vi "SentinelController v33.vi"() -> ()   [LabVIEW 2011] (continued)
                                n1247 = local write "SC handler states hid"(SC_handler_states."responding to serial poll" ("SC Test Interface States")) -> ()
                                }
                                }
                                }
                                }
                              }
                              frame "reading" {
                                n1248 = flat-sequence {
                                tunnel: [w1473] -> w1470
                                tunnel: w1470 -> [w1486]
                                tunnel: [w1486] -> w1469
                                tunnel: w1469 -> [w1489]
                                tunnel: [w1488] -> w1468
                                tunnel: w1468 -> [w1490]
                                frame #0 {
                                n1249 = local read "VISA bus 0 resource name out hid"() -> (w1479:refnum<visa-resource-name>)
                                n1250 = local read "VISA bus 0 error out hid"() -> (w1480:errorcluster)
                                n1251 = local read "GPIB Bus 0 traffic"() -> (w1477:string)
                                n1252 = VISA Read(VISA resource name=w1479, byte count=256, error in (no error)=w1480) -> (VISA resource name out=w1478:refnum<visa-resource-name>, read buffer=w1473:string, error out=w1481:errorcluster)  [unwired: 1 out]
                                n1253 = String Subset(string=w1473, length (rest)=1 ("length (rest)")) -> ()  [unwired: 1 in, 1 out]
                                n1254 = local write "VISA bus 0 resource name out hid"(w1478) -> ()
                                n1255 = local write "Message from tester hid"(w1473) -> ()
                                n1256 = Unbundle By Name(w1481) -> ("status"=w1484:bool)
                                n1257 = Concatenate Strings(w1477, "\r\n", "Bus 0 read: " ("string"), w1473) -> (w1475:string)
                                n1258 = local write "GPIB Bus 0 traffic"(w1475) -> ()
                                n1259 = local write "GPIB bus 0 read error"(w1484) -> ()
                                }
                                frame #1 {
                                n1260 = local read "Slow for  Diagnostics"() -> (w1485:bool)
                                n1261 = case shown="True" w1485 {
                                frame False {
                                }
                                frame True {
                                n1262 = local read "GPIB wait time (ms)"() -> (w1487:u32)
                                n1263 = Wait (ms)(milliseconds to wait=w1487) -> ()  [unwired: 1 out]
                                }
                                }
                                }
                                frame #2 {
                                n1264 = call <vilib>:"Trim Whitespace.vi"("string"=w1489) -> ("trimmed string"=w1488:string)  [unwired: 1 in]
                                }
                                frame #3 {
                                n1265 = Match Pattern(string=w1490, regular expression="?") -> (offset past match=w1493:i32)  [unwired: 1 in, 3 out]
                                n1266 = Greater Or Equal To 0?(x=w1493) -> (x >= 0?=w1491:bool)
                                n1267 = case shown="False" w1491 {
                                tunnel: w1490 -> [w1497 w1512]
                                frame False {
                                n1268 = Match Pattern(string=w1497, regular expression=":" ("true string")) -> (offset past match=w1494:i32)  [unwired: 1 in, 3 out]
                                n1269 = Greater Or Equal To 0?(x=w1494) -> (x >= 0?=w1495:bool)
                                n1270 = case shown="False" w1495 {
                                tunnel: w1497 -> [w1500 w1507]
                                frame False {
                                n1271 = call <vilib>:"Space Constant.vi"() -> ("String"=w1501:string)
                                n1272 = Match Pattern(string=w1500, regular expression=w1501) -> (offset past match=w1499:i32)  [unwired: 1 in, 3 out]
                                n1273 = Greater Or Equal To 0?(x=w1499) -> (x >= 0?=w1498:bool)
                                n1274 = case shown="False" w1498 {
                                tunnel: w1500 -> [w1502 w1504]
                                frame False {
                                n1275 = local write "GPIB parsed msg from tester hid"(w1502) -> ()
                                }
                                frame True {
                                n1276 = call <vilib>:"Space Constant.vi"() -> ("String"=w1505:string)
                                n1277 = Match Pattern(string=w1504, regular expression=w1505) -> (before substring=w1503:string)  [unwired: 1 in, 3 out]
                                n1278 = local write "GPIB parsed msg from tester hid"(w1503) -> ()
                                }
                                }
                                }
                                frame True {
                                n1279 = Match Pattern(string=w1507, regular expression=":") -> (before substring=w1506:string)  [unwired: 1 in, 3 out]
                                n1280 = local write "GPIB parsed msg from tester hid"(w1506) -> ()
                                }
                                }
                                }
                                frame True {
                                w1510 = "?" ("regular expression")
                                n1281 = Match Pattern(string=w1512, regular expression=w1510) -> (before substring=w1511:string)  [unwired: 1 in, 3 out]
                                n1282 = Concatenate Strings(w1511, w1510) -> (w1509:string)
                                n1283 = local write "GPIB parsed msg from tester hid"(w1509) -> ()
                                }
                                }
                                }
                                frame #4 {
                                n1284 = local read "GPIB parsed msg from tester hid"() -> (w1513:string)
                                n1285 = case shown="\"Fullsites?\"" w1513 {
                                frame "SQR" {
                                n1286 = local write "SC handler states hid"(SC_handler_states."responding to SRQ" ("SC Test Interface States")) -> ()
                                }
                                frame "*IDN?" {
                                n1287 = local write "SC handler states hid"(SC_handler_states."responding to *IDN?" ("SC Test Interface States")) -> ()
                                }
                                frame "FR?" {
                                n1288 = local write "SC handler states hid"(SC_handler_states."responding to FR?" ("SC Test Interface States")) -> ()
                                }
                                frame "*STB?" {
                                n1289 = local write "SC handler states hid"(SC_handler_states."responding to serial poll" ("SC Test Interface States")) -> ()
                                }
                                frame "SITES?" {
                                n1290 = local read "Tester online"() -> (w1520:bool)
                                n1291 = local read "POWER"() -> (w1518:bool)
                                n1292 = Compound Arithmetic op=AND(w1520, w1518) -> (w1519:bool)
                                n1293 = case shown="True" w1519 {
                                frame False {
                                n1294 = local write "SC handler states hid"(SC_handler_states."closing bus" ("SC virtual handler states")) -> ()
                                }
                                frame True {
                                n1295 = flat-sequence {
                                frame #0 {
                                n1296 = while {
                                stop <- w1523 stop-if-true
                                n1297 = local read "H1 Ready with sites"() -> (w1525:bool)
                                n1298 = local read "H2 Ready with sites"() -> (w1524:bool)
                                n1299 = Or(x=w1525, y=w1524) -> (x .or. y?=w1523:bool)
                                n1300 = Wait (ms)(milliseconds to wait=u32 5) -> ()  [unwired: 1 out]
                                }
                                }
                                frame #1 {
                                n1301 = local write "SC handler states hid"(SC_handler_states."responding to serial poll" ("SC Test Interface States")) -> ()
                                }
                                }
                                }
                                }
                                }
                                frame "Fullsites?" {
                                n1302 = local read "Tester online"() -> (w1529:bool)
                                n1303 = local read "POWER"() -> (w1527:bool)
                                n1304 = Compound Arithmetic op=AND(w1529, w1527) -> (w1528:bool)
                                n1305 = case shown="True" w1528 {
                                frame False {
                                n1306 = local write "SC handler states hid"(SC_handler_states."closing bus" ("SC virtual handler states")) -> ()
                                }
                                frame True {
                                n1307 = flat-sequence {
                                frame #0 {
                                n1308 = while {
                                stop <- w1532 stop-if-true
                                n1309 = local read "H1 Lock"() -> (w1534:bool)
                                n1310 = local read "H2 Lock"() -> (w1533:bool)
                                n1311 = Or(x=w1534, y=w1533) -> (x .or. y?=w1532:bool)
                                n1312 = Wait (ms)(milliseconds to wait=u32 5) -> ()  [unwired: 1 out]
                                }
                                }
                                frame #1 {
                                n1313 = local write "SC handler states hid"(SC_handler_states."responding to Fullsites?" ("SC Test Interface States")) -> ()
                                }
                                }
                                }
                                }
                                }
                                frame "HIDN?" {
                                n1314 = local write "SC handler states hid"(SC_handler_states."responding to HIDN?" ("SC Test Interface States")) -> ()
                                }
                                frame "HAND?" {
                                n1315 = local write "SC handler states hid"(SC_handler_states."respond to HAND?" ("SC Test Interface States")) -> ()
                                }
                                frame "A BIN" {
                                n1316 = flat-sequence {
                                frame #0 {
                                n1317 = local read "Message from tester hid"() -> (w1538:string)
                                n1318 = local write "Binning string from tester hid"(w1538) -> ()
                                }
                                frame #1 {
                                n1319 = local write "SC handler states hid"(SC_handler_states."responding to HIDN?" ("SC Test Interface States")) -> ()
                                }
                                }
                                }
                                frame "BINON" {
                                # "THis may need to be handler specific (lock dependent)"
                                n1320 = flat-sequence {
                                frame #0 {
                                n1321 = local read "Message from tester hid"() -> (w1540:string)
                                n1322 = local write "Binning string from tester hid"(w1540) -> ()
                                }
                                frame #1 {
                                n1323 = local write "SC handler states hid"(SC_handler_states."responding to BINON" ("SC Test Interface States")) -> ()
                                }
                                }
                                }
                                frame "ECHOOK" {
                                n1324 = local write "SC handler states hid"(SC_handler_states."responding to ECHOOK" ("SC Test Interface States")) -> ()
                                }
                                frame "ECHONG" {
                                n1325 = local write "SC handler states hid"(SC_handler_states."responding to ECHONG" ("SC Test Interface States")) -> ()
                                }
                                frame Default {
                                n1326 = local write "SC handler states hid"(SC_handler_states."waiting on event" ("SC Test Interface States")) -> ()
                                }
                                }
                                }
                                }
                              }
                              frame "responding to *IDN?" {
                                n1327 = flat-sequence {
                                frame #0 {
                                n1328 = while {
                                stop <- w1548 stop-if-true
                                w1550 = "Sentinel Controller Handler Interface"
                                n1329 = local read "VISA bus 0 resource name out hid"() -> (w1558:refnum<visa-resource-name>)
                                n1330 = local read "VISA bus 0 error out hid"() -> (w1557:errorcluster)
                                n1331 = local read "GPIB Bus 0 traffic"() -> (w1554:string)
                                n1332 = VISA Write(VISA resource name=w1558, write buffer=w1550, error in (no error)=w1557) -> (VISA resource name out=w1556:refnum<visa-resource-name>, return count=w1549:u32, error out=w1555:errorcluster)
                                n1333 = local write "VISA bus 0 resource name out hid"(w1556) -> ()
                                n1334 = local write "VISA bus 0 error out hid"(w1555) -> ()
                                n1335 = Unbundle By Name(w1555) -> ("status"=w1547:bool)
                                n1336 = Concatenate Strings(w1554, "\r\n", "Bus 0 write: " ("string"), w1550) -> (w1552:string)
                                n1337 = Greater Than 0?(x=w1549) -> (x > 0?=w1548:bool)
                                n1338 = local write "GPIB bus 0 write error"(w1547) -> ()
                                n1339 = local write "GPIB Bus 0 traffic"(w1552) -> ()
                                }
                                }
                                frame #1 {
                                n1340 = local write "SC handler states hid"(SC_handler_states."waiting on event" ("SC Test Interface States")) -> ()
                                }
                                }
                              }
                              frame "responding to SRQ" {
                                n1341 = flat-sequence {
                                frame #0 {
                                n1342 = local read "GPIB Bus 0 traffic"() -> (w1566:string)
                                n1343 = Concatenate Strings(w1566, "\r\n", "Bus 0 write: " ("string"), "Responding to \"SRQ MASK 65\" from tester.\nThis message is sent to NS6040 handlers every cycle.\nNo response back to tester.") -> (w1564:string)
                                n1344 = local write "GPIB Bus 0 traffic"(w1564) -> ()
                                }
                                frame #1 {
                                n1345 = local write "SC handler states hid"(SC_handler_states."waiting on event" ("SC Test Interface States")) -> ()
                                }
                                }
                              }
                              frame "respond to HAND?" {
                                n1346 = local read "H1 Lock"() -> (w1570:bool)
                                n1347 = case shown="False" w1570 {
                                frame False {
                                n1348 = local read "H2 Lock"() -> (w1571:bool)
                                n1349 = case shown="True" w1571 {
                                frame False {
                                n1350 = flat-sequence {
                                frame #0 {
                                n1351 = One Button Dialog(message="Fatal error 200:\nThe SC responded to a handler being ready with devices\nto test, but when the SC check for a lock when responding\nto *HAND?, no handler had a lock. \nPlease report this bug to Celerint at www.celerint.com  ") -> ()  [unwired: 1 in, 1 out]
                                }
                                frame #1 {
                                n1352 = local write "SC handler states hid"(SC_handler_states."closing bus" ("SC Test Interface States")) -> ()
                                }
                                }
                                }
                                frame True {
                                n1353 = flat-sequence {
                                frame #0 {
                                n1354 = while {
                                stop <- w1575 stop-if-true
                                w1576 = "H2" ("string")
                                n1355 = local read "VISA bus 0 resource name out hid"() -> (w1582:refnum<visa-resource-name>)
                                n1356 = local read "GPIB Bus 0 traffic"() -> (w1580:string)
                                n1357 = local read "VISA bus 0 error out hid"() -> (w1581:errorcluster)
                                n1358 = Concatenate Strings(w1580, "\r\n", "H2: Bus 0 write: " ("string"), w1576) -> (w1578:string)
                                n1359 = VISA Write(VISA resource name=w1582, write buffer=w1576, error in (no error)=w1581) -> (VISA resource name out=w1583:refnum<visa-resource-name>, return count=w1574:u32, error out=w1584:errorcluster)
                                n1360 = local write "VISA bus 0 error out hid"(w1584) -> ()
                                n1361 = Unbundle By Name(w1584) -> ("status"=w1585:bool)
                                n1362 = local write "GPIB Bus 0 traffic"(w1578) -> ()
                                n1363 = Greater Than 0?(x=w1574) -> (x > 0?=w1575:bool)
                                n1364 = local write "VISA bus 0 resource name out hid"(w1583) -> ()
                                n1365 = local write "GPIB bus 0 write error"(w1585) -> ()
                                }
                                }
                                frame #1 {
                                n1366 = local write "SC handler states hid"(SC_handler_states."waiting on event" ("SC Test Interface States")) -> ()
                                }
                                }
                                }
                                }
                                }
                                frame True {
                                n1367 = flat-sequence {
                                frame #0 {
                                n1368 = while {
                                stop <- w1588 stop-if-true
                                w1589 = "H1" ("string")
                                n1369 = local read "VISA bus 0 resource name out hid"() -> (w1595:refnum<visa-resource-name>)
                                n1370 = local read "GPIB Bus 0 traffic"() -> (w1593:string)
                                n1371 = local read "VISA bus 0 error out hid"() -> (w1594:errorcluster)
                                n1372 = Concatenate Strings(w1593, "\r\n", "H1: Bus 0 write: " ("string"), w1589) -> (w1591:string)
                                n1373 = VISA Write(VISA resource name=w1595, write buffer=w1589, error in (no error)=w1594) -> (VISA resource name out=w1596:refnum<visa-resource-name>, return count=w1587:u32, error out=w1597:errorcluster)
                                n1374 = local write "VISA bus 0 resource name out hid"(w1596) -> ()
                                n1375 = local write "VISA bus 0 error out hid"(w1597) -> ()
                                n1376 = Unbundle By Name(w1597) -> ("status"=w1598:bool)
                                n1377 = local write "GPIB Bus 0 traffic"(w1591) -> ()
                                n1378 = Greater Than 0?(x=w1587) -> (x > 0?=w1588:bool)
                                n1379 = local write "GPIB bus 0 write error"(w1598) -> ()
                                }
                                }
                                frame #1 {
                                n1380 = local write "SC handler states hid"(SC_handler_states."waiting on event" ("SC Test Interface States")) -> ()
                                }
                                }
                                }
                                }
                              }
                              frame "responding to HIDN?" {
                                n1381 = local read "H1 Lock"() -> (w1602:bool)
                                n1382 = case shown="False" w1602 {
                                frame False {
                                n1383 = local read "H2 Lock"() -> (w1603:bool)
                                n1384 = case shown="True" w1603 {
                                frame False {
                                n1385 = flat-sequence {
                                frame #0 {
                                n1386 = One Button Dialog(message="Fatal error 201:\nThe SC responded to a handler being ready with devices\nto test, but when the SC check for a lock when responding\nto *HIDN?, no handler had a lock. \nPlease report this bug to Celerint at www.celerint.com  ") -> ()  [unwired: 1 in, 1 out]
                                }
                                frame #1 {
                                n1387 = local write "SC handler states hid"(SC_handler_states."testing" ("SC Test Interface States")) -> ()
                                }
                                }
                                }
                                frame True {
                                n1388 = flat-sequence {
                                frame #0 {
                                n1389 = while {
                                stop <- w1607 stop-if-true
                                n1390 = local read "VISA bus 0 resource name out hid"() -> (w1614:refnum<visa-resource-name>)
                                n1391 = local read "H2 response to *HAND? hid"() -> (w1608:string)
                                n1392 = local read "VISA bus 0 error out hid"() -> (w1613:errorcluster)
                                n1393 = local read "GPIB Bus 0 traffic"() -> (w1612:string)
                                n1394 = VISA Write(VISA resource name=w1614, write buffer=w1608, error in (no error)=w1613) -> (VISA resource name out=w1615:refnum<visa-resource-name>, return count=w1606:u32, error out=w1616:errorcluster)
                                n1395 = local write "VISA bus 0 error out hid"(w1616) -> ()
                                n1396 = Unbundle By Name(w1616) -> ("status"=w1617:bool)
                                n1397 = Concatenate Strings(w1612, "\r\n", "H2: Bus 0 write: " ("string"), w1608) -> (w1610:string)
                                n1398 = Greater Than 0?(x=w1606) -> (x > 0?=w1607:bool)
                                n1399 = local write "VISA bus 0 resource name out hid"(w1615) -> ()
                                n1400 = local write "GPIB Bus 0 traffic"(w1610) -> ()
                                n1401 = local write "GPIB bus 0 write error"(w1617) -> ()
                                }
                                }
                                frame #1 {
                                n1402 = local write "SC handler states hid"(SC_handler_states."waiting on event" ("SC Test Interface States")) -> ()
                                }
                                }
                                }
                                }
                                }
                                frame True {
                                n1403 = flat-sequence {
                                frame #0 {
                                n1404 = while {
                                stop <- w1620 stop-if-true
                                n1405 = local read "VISA bus 0 resource name out hid"() -> (w1627:refnum<visa-resource-name>)
                                n1406 = local read "H1 response to *HAND? hid"() -> (w1621:string)
                                n1407 = local read "VISA bus 0 error out hid"() -> (w1626:errorcluster)
                                n1408 = local read "GPIB Bus 0 traffic"() -> (w1625:string)
                                n1409 = VISA Write(VISA resource name=w1627, write buffer=w1621, error in (no error)=w1626) -> (VISA resource name out=w1628:refnum<visa-resource-name>, return count=w1619:u32, error out=w1629:errorcluster)
                                n1410 = local write "VISA bus 0 resource name out hid"(w1628) -> ()
                                n1411 = local write "VISA bus 0 error out hid"(w1629) -> ()
                                n1412 = Unbundle By Name(w1629) -> ("status"=w1630:bool)
                                n1413 = Concatenate Strings(w1625, "\r\n", "H1: Bus 0 write: " ("string"), w1621) -> (w1623:string)
                                n1414 = Greater Than 0?(x=w1619) -> (x > 0?=w1620:bool)
                                n1415 = local write "GPIB Bus 0 traffic"(w1623) -> ()
                                n1416 = local write "GPIB bus 0 write error"(w1630) -> ()
                                }
                                }
                                frame #1 {
                                n1417 = local write "SC handler states hid"(SC_handler_states."waiting on event" ("SC Test Interface States")) -> ()
                                }
                                }
                                }
                                }
                              }
                              frame "responding to FR?" {
                                n1418 = flat-sequence {
                                frame #0 {
                                n1419 = local read "H1 Ready with sites"() -> (w1634:bool)
                                n1420 = local read "H2 Ready with sites"() -> (w1635:bool)
                                n1421 = Or(x=w1634, y=w1635) -> (x .or. y?=w1636:bool)
                                n1422 = case shown="True" w1636 {
                                frame False {
                                n1423 = flat-sequence {
                                frame #0 {
                                n1424 = while {
                                stop <- w1637 stop-if-true
                                n1425 = Wait (ms)(milliseconds to wait=u32 100) -> ()  [unwired: 1 out]
                                n1426 = One Button Dialog(message="Error in state \"responding to FR?.\nA handler should have been ready,\nbut none was set \"Ready with sites.\"\nClosing Bus 0.") -> (true=w1637:bool)  [unwired: 1 in]
                                }
                                }
                                frame #1 {
                                n1427 = local write "SC handler states hid"(SC_handler_states."closing bus" ("SC Test Interface States")) -> ()
                                }
                                }
                                }
                                frame True {
                                n1428 = while {
                                stop <- w1642 stop-if-true
                                w1644 = "FR0"
                                n1429 = local read "VISA bus 0 resource name out hid"() -> (w1652:refnum<visa-resource-name>)
                                n1430 = local read "VISA bus 0 error out hid"() -> (w1651:errorcluster)
                                n1431 = local read "GPIB Bus 0 traffic"() -> (w1648:string)
                                n1432 = VISA Write(VISA resource name=w1652, write buffer=w1644, error in (no error)=w1651) -> (VISA resource name out=w1650:refnum<visa-resource-name>, return count=w1643:u32, error out=w1649:errorcluster)
                                n1433 = local write "VISA bus 0 resource name out hid"(w1650) -> ()
                                n1434 = local write "VISA bus 0 error out hid"(w1649) -> ()
                                n1435 = Unbundle By Name(w1649) -> ("status"=w1641:bool)
                                n1436 = Concatenate Strings(w1648, "\r\n", "Bus 0 write: " ("string"), w1644) -> (w1646:string)
                                n1437 = Greater Than 0?(x=w1643) -> (x > 0?=w1642:bool)
                                n1438 = local write "GPIB bus 0 write error"(w1641) -> ()
                                n1439 = local write "GPIB Bus 0 traffic"(w1646) -> ()
                                }
                                }
                                }
                                }
                                frame #1 {
                                n1440 = local write "SC handler states hid"(SC_handler_states."waiting on event" ("SC Test Interface States")) -> ()
                                }
                                }
                              }
                              frame "responding to serial poll" {
                                n1441 = flat-sequence {
                                frame #0 {
                                # "This is the engine that decides if H1 is checked first or H2"
                                n1442 = local read "GPIB Bus 0 traffic"() -> (w1660:string)
                                n1443 = Concatenate Strings(w1660, "\r\n", "Bus 0 write: " ("string"), "Responding to Serial Poll from tester.\nSTB was set to 0100 0001 and should now be reset to 0000 0000\nA handler is ready. ") -> (w1658:string)
                                n1444 = local write "GPIB Bus 0 traffic"(w1658) -> ()
                                }
                                frame #1 {
                                n1445 = flat-sequence {
                                frame #0 {
                                n1446 = local read "Last locked handler hid"() -> (w1661:enum16{"H1", "H2"})
                                n1447 = case shown="\"H2\"" w1661 {
                                frame "H1", Default {
                                n1448 = local read "H2 Ready with sites"() -> (w1662:bool)
                                n1449 = case shown="False" w1662 {
                                frame False {
                                n1450 = local read "H1 Ready with sites"() -> (w1663:bool)
                                n1451 = case shown="True" w1663 {
                                frame False {
                                # "end up here only if neither handler is waiting and ready"
                                }
                                frame True {
                                n1452 = flat-sequence {
                                frame #0 {
                                n1453 = local write "H2 Lock"(FALSE ("H1 Lock")) -> ()
                                n1454 = local write "H1 Lock"(TRUE ("H1 Lock")) -> ()
                                n1455 = local write "Last locked handler hid"(enum16{"H1", "H2"}."H1" ("Last locked handler")) -> ()
                                }
                                frame #1 {
                                n1456 = local read "H1 loop counter hid"() -> (w1668:u32)
                                n1457 = Increment(x=w1668) -> (x+1=w1667:u32)
                                n1458 = local write "H1 loop counter hid"(w1667) -> ()
                                }
                                }
                                }
                                }
                                }
                                frame True {
                                n1459 = flat-sequence {
                                frame #0 {
                                n1460 = local write "H1 Lock"(FALSE ("H1 Lock")) -> ()
                                n1461 = local write "H2 Lock"(TRUE ("H1 Lock")) -> ()
                                n1462 = local write "Last locked handler hid"(enum16{"H1", "H2"}."H2" ("Last locked handler")) -> ()
                                }
                                frame #1 {
                                n1463 = local read "H2 loop counter hid"() -> (w1672:u32)
                                n1464 = Increment(x=w1672) -> (x+1=w1673:u32)
                                n1465 = local write "H2 loop counter hid"(w1673) -> ()
                                }
                                }
                                }
                                }
                                }
                                frame "H2" {
                                n1466 = local read "H1 Ready with sites"() -> (w1674:bool)
                                n1467 = case shown="True" w1674 {
                                frame False {
                                n1468 = local read "H2 Ready with sites"() -> (w1675:bool)
                                n1469 = case shown="True" w1675 {
                                frame False {
                                # "end up here only if neither handler is waiting and ready"
                                }
                                frame True {
                                n1470 = flat-sequence {
                                frame #0 {
                                n1471 = local write "H2 Lock"(TRUE ("H1 Lock")) -> ()
                                n1472 = local write "H1 Lock"(FALSE ("H1 Lock")) -> ()
                                n1473 = local write "Last locked handler hid"(enum16{"H1", "H2"}."H2" ("Last locked handler")) -> ()
                                }
                                frame #1 {
                                n1474 = local read "H2 loop counter hid"() -> (w1679:u32)
                                n1475 = Increment(x=w1679) -> (x+1=w1680:u32)
                                n1476 = local write "H2 loop counter hid"(w1680) -> ()
                                }
                                }
                                }
                                }
                                }
                                frame True {
                                n1477 = flat-sequence {
                                frame #0 {
                                n1478 = local write "H1 Lock"(TRUE ("H1 Lock")) -> ()
                                n1479 = local write "H2 Lock"(FALSE ("H1 Lock")) -> ()
                                n1480 = local write "Last locked handler hid"(enum16{"H1", "H2"}."H1" ("Last locked handler")) -> ()
                                }
                                frame #1 {
                                n1481 = local read "H1 loop counter hid"() -> (w1685:u32)
                                n1482 = Increment(x=w1685) -> (x+1=w1684:u32)
                                n1483 = local write "H1 loop counter hid"(w1684) -> ()
                                }
                                }
                                }
                                }
                                }
                                }
                                }
                                frame #1 {
                                n1484 = local write "SC handler states hid"(SC_handler_states."waiting on event" ("SC Test Interface States")) -> ()
                                }
                                }
                                }
                                }
                              }
                              frame "responding to Fullsites?" {
                                n1485 = local read "H1 Ready with sites"() -> (w1687:bool)
                                n1486 = local read "H2 Ready with sites"() -> (w1688:bool)
                                n1487 = Or(x=w1687, y=w1688) -> (x .or. y?=w1693:bool)
                                n1488 = case shown="True" w1693 {
                                tunnel: w1692 -> [w1694 w1708]
                                tunnel: w1691 -> [w1695 w1707]
                                tunnel: [w1694 w1701] -> w1690
                                tunnel: [w1695 w1704] -> w1689
                                frame False {
                                n1489 = local write "SC handler states hid"(SC_handler_states."waiting on event" ("SC Test Interface States")) -> ()
                                }
                                frame True {
                                n1490 = flat-sequence {
                                tunnel: w1707 -> [w1711]
                                tunnel: w1708 -> [w1712]
                                tunnel: [w1710] -> w1706
                                tunnel: [w1709] -> w1703
                                tunnel: w1706 -> [w1725]
                                tunnel: [w1725] -> w1705
                                tunnel: w1703 -> [w1724]
                                tunnel: [w1724] -> w1702
                                tunnel: w1705 -> [w1787]
                                tunnel: w1702 -> [w1786]
                                tunnel: [w1787] -> w1700
                                tunnel: [w1786] -> w1699
                                tunnel: w1700 -> [w1796]
                                tunnel: w1699 -> [w1795]
                                tunnel: [w1796] -> w1698
                                tunnel: [w1795] -> w1697
                                tunnel: [w1798] -> w1701
                                tunnel: [w1799] -> w1704
                                tunnel: w1698 -> [w1799]
                                tunnel: w1697 -> [w1798]
                                frame #0 {
                                n1491 = local read "SC measured test time hid"() -> (w1713:dbl)
                                n1492 = local read "SC measured wait time hid"() -> (w1714:dbl)
                                n1493 = Add(x=w1713, y=w1714) -> (x+y=w1720:dbl)
                                n1494 = local read "Tester loop counter hid"() -> (w1716:u32)
                                n1495 = local read "Utilization averaging"() -> (w1715:i32)
                                n1496 = Divide(x=w1713, y=w1720) -> (x/y=w1721:dbl)
                                n1497 = Multiply(x=100.0, y=w1721) -> (x*y=w1717:dbl)
                                n1498 = call "moving_avg_core.vi"("Array in"=w1711, "avg"=w1715, "accumulator in"=w1712, "i"=w1716, "data in"=w1717) -> ("Array out"=w1710:dbl[], "accumulator out"=w1709:dbl, "rolling avg out"=w1718:dbl)  [unwired: 4 in]
                                n1499 = local write "Sys utilization"(w1718) -> ()
                                n1500 = Bundle(w1717, "rolling avg out"=w1718) -> (w1719:cluster{dbl, "rolling avg out":dbl})  [unwired: 1 in]
                                n1501 = local write "SysUtilMon"(w1719) -> ()
                                }
                                frame #1 {
                                n1502 = local read "Last locked handler hid"() -> (w1723:enum16{"H1", "H2"})
                                n1503 = case shown="\"H2\"" w1723 {
                                frame "H1", Default {
                                n1504 = local read "H2 Ready with sites"() -> (w1726:bool)
                                n1505 = case shown="False" w1726 {
                                frame False {
                                n1506 = local read "H1 Ready with sites"() -> (w1727:bool)
                                n1507 = case shown="True" w1727 {
                                frame False {
                                # "end up here only if neither handler is waiting and ready"
                                }
                                frame True {
                                n1508 = flat-sequence {
                                frame #0 {
                                n1509 = while {
                                stop <- w1728 stop-if-true
                                n1510 = local read "VISA bus 0 resource name out hid"() -> (w1737:refnum<visa-resource-name>)
                                n1511 = local read "H1 FULLSITES? response hid"() -> (w1731:string)
                                n1512 = local read "VISA bus 0 error out hid"() -> (w1738:errorcluster)
                                n1513 = VISA Write(VISA resource name=w1737, write buffer=w1731, error in (no error)=w1738) -> (VISA resource name out=w1736:refnum<visa-resource-name>, return count=w1729:u32, error out=w1735:errorcluster)
                                n1514 = local write "VISA bus 0 resource name out hid"(w1736) -> ()
                                n1515 = Unbundle By Name(w1735) -> ("status"=w1739:bool)
                                n1516 = local write "VISA bus 0 error out hid"(w1735) -> ()
                                n1517 = Concatenate Strings("H1: Tester test cycle start" ("string"), "\r\n", "Bus 0 write: " ("string"), w1731) -> (w1733:string)
                                n1518 = Greater Than 0?(x=w1729) -> (x > 0?=w1728:bool)
                                n1519 = local write "GPIB Bus 0 traffic"(w1733) -> ()
                                n1520 = local write "GPIB bus 0 write error"(w1739) -> ()
                                }
                                }
                                frame #1 {
                                n1521 = local read "H1 loop counter hid"() -> (w1741:u32)
                                n1522 = Increment(x=w1741) -> (x+1=w1740:u32)
                                n1523 = local write "H1 loop counter hid"(w1740) -> ()
                                }
                                }
                                }
                                }
                                }
                                frame True {
                                n1524 = flat-sequence {
                                frame #0 {
                                n1525 = while {
                                stop <- w1743 stop-if-true
                                n1526 = local read "VISA bus 0 resource name out hid"() -> (w1751:refnum<visa-resource-name>)
                                n1527 = local read "H2 FULLSITES? response hid"() -> (w1745:string)
                                n1528 = local read "VISA bus 0 error out hid"() -> (w1752:errorcluster)
                                n1529 = VISA Write(VISA resource name=w1751, write buffer=w1745, error in (no error)=w1752) -> (VISA resource name out=w1750:refnum<visa-resource-name>, return count=w1742:u32, error out=w1749:errorcluster)
                                n1530 = local write "VISA bus 0 resource name out hid"(w1750) -> ()
                                n1531 = Unbundle By Name(w1749) -> ("status"=w1753:bool)
                                n1532 = local write "VISA bus 0 error out hid"(w1749) -> ()
                                n1533 = Concatenate Strings("H2: Tester test cycle start" ("string"), "\r\n", "Bus 0 write: " ("string"), w1745) -> (w1747:string)
                                n1534 = Greater Than 0?(x=w1742) -> (x > 0?=w1743:bool)
                                n1535 = local write "GPIB Bus 0 traffic"(w1747) -> ()
                                n1536 = local write "GPIB bus 0 write error"(w1753) -> ()
                                }
                                }
                                frame #1 {
                                n1537 = local read "H2 loop counter hid"() -> (w1754:u32)
                                n1538 = Increment(x=w1754) -> (x+1=w1755:u32)
                                n1539 = local write "H2 loop counter hid"(w1755) -> ()
                                }
                                }
                                }
                                }
                                }
                                frame "H2" {
                                n1540 = local read "H1 Ready with sites"() -> (w1756:bool)
                                n1541 = case shown="True" w1756 {
                                frame False {
                                n1542 = local read "H2 Ready with sites"() -> (w1757:bool)
                                n1543 = case shown="True" w1757 {
                                frame False {
                                # "end up here only if neither handler is waiting and ready"
                                }
                                frame True {
                                n1544 = flat-sequence {
                                frame #0 {
                                n1545 = while {
                                stop <- w1759 stop-if-true
                                n1546 = local read "VISA bus 0 resource name out hid"() -> (w1767:refnum<visa-resource-name>)
                                n1547 = local read "H2 FULLSITES? response hid"() -> (w1761:string)
                                n1548 = local read "VISA bus 0 error out hid"() -> (w1768:errorcluster)
                                n1549 = VISA Write(VISA resource name=w1767, write buffer=w1761, error in (no error)=w1768) -> (VISA resource name out=w1766:refnum<visa-resource-name>, return count=w1758:u32, error out=w1765:errorcluster)
                                n1550 = local write "VISA bus 0 resource name out hid"(w1766) -> ()
                                n1551 = Unbundle By Name(w1765) -> ("status"=w1769:bool)
                                n1552 = local write "VISA bus 0 error out hid"(w1765) -> ()
                                n1553 = Concatenate Strings("H2: Tester test cycle start" ("string"), "\r\n", "Bus 0 write: " ("string"), w1761) -> (w1763:string)
                                n1554 = Greater Than 0?(x=w1758) -> (x > 0?=w1759:bool)
                                n1555 = local write "GPIB Bus 0 traffic"(w1763) -> ()
                                n1556 = local write "GPIB bus 0 write error"(w1769) -> ()
                                }
                                }
                                frame #1 {
                                n1557 = local read "H2 loop counter hid"() -> (w1770:u32)
                                n1558 = Increment(x=w1770) -> (x+1=w1771:u32)
                                n1559 = local write "H2 loop counter hid"(w1771) -> ()
                                }
                                }
                                }
                                }
                                }
                                frame True {
                                n1560 = flat-sequence {
                                frame #0 {
                                n1561 = while {
                                stop <- w1772 stop-if-true
                                n1562 = local read "VISA bus 0 resource name out hid"() -> (w1781:refnum<visa-resource-name>)
                                n1563 = local read "H1 FULLSITES? response hid"() -> (w1775:string)
                                n1564 = local read "VISA bus 0 error out hid"() -> (w1782:errorcluster)
                                n1565 = VISA Write(VISA resource name=w1781, write buffer=w1775, error in (no error)=w1782) -> (VISA resource name out=w1780:refnum<visa-resource-name>, return count=w1773:u32, error out=w1779:errorcluster)
                                n1566 = local write "VISA bus 0 resource name out hid"(w1780) -> ()
                                n1567 = Unbundle By Name(w1779) -> ("status"=w1783:bool)
                                n1568 = local write "VISA bus 0 error out hid"(w1779) -> ()
                                n1569 = Concatenate Strings("H1: Tester test cycle start" ("string"), "\r\n", "Bus 0 write: " ("string"), w1775) -> (w1777:string)
                                n1570 = Greater Than 0?(x=w1773) -> (x > 0?=w1772:bool)
                                n1571 = local write "GPIB Bus 0 traffic"(w1777) -> ()
                                n1572 = local write "GPIB bus 0 write error"(w1783) -> ()
                                }
                                }
                                frame #1 {
                                n1573 = local read "H1 loop counter hid"() -> (w1785:u32)
                                n1574 = Increment(x=w1785) -> (x+1=w1784:u32)
                                n1575 = local write "H1 loop counter hid"(w1784) -> ()
                                }
                                }
                                }
                                }
                                }
                                }
                                }
                                frame #2 {
                                n1576 = Tick Count (ms)() -> (millisecond timer value=w1788:u32)
                                n1577 = Tick Count (ms)() -> (millisecond timer value=w1789:u32)
                                n1578 = local write "tester tt start hid"(w1788) -> ()
                                n1579 = local write "tester wt end hid"(w1789) -> ()
                                }
                                frame #3 {
                                n1580 = local read "tester wt start hid"() -> (w1793:u32)
                                n1581 = local read "tester wt end hid"() -> (w1794:u32)
                                n1582 = Subtract(x=w1794, y=w1793) -> (x-y=w1792:u32)
                                n1583 = Divide(x=w1792, y=u32 1000) -> (x/y=w1790:dbl)
                                n1584 = local write "SC measured wait time hid"(w1790) -> ()
                                }
                                frame #4 {
                                n1585 = local write "SC handler states hid"(SC_handler_states."testing" ("SC Test Interface States")) -> ()
                                }
                                }
                                }
                                }
                              }
                              frame "responding to SITES?" {
                                n1586 = local read "H1 Ready with sites"() -> (w1800:bool)
                                n1587 = local read "H2 Ready with sites"() -> (w1801:bool)
                                n1588 = Or(x=w1800, y=w1801) -> (x .or. y?=w1806:bool)
                                n1589 = case shown="True" w1806 {
                                tunnel: w1805 -> [w1807 w1821]
                                tunnel: w1804 -> [w1808 w1820]
                                tunnel: [w1807 w1814] -> w1803
                                tunnel: [w1808 w1817] -> w1802
                                frame False {
                                n1590 = local write "SC handler states hid"(SC_handler_states."waiting on event" ("SC Test Interface States")) -> ()
                                }
                                frame True {
                                n1591 = flat-sequence {
                                tunnel: w1820 -> [w1824]
                                tunnel: w1821 -> [w1825]
                                tunnel: [w1823] -> w1819
                                tunnel: [w1822] -> w1816
                                tunnel: w1819 -> [w1838]
                                tunnel: [w1838] -> w1818
                                tunnel: w1816 -> [w1837]
                                tunnel: [w1837] -> w1815
                                tunnel: w1818 -> [w1910]
                                tunnel: w1815 -> [w1909]
                                tunnel: [w1910] -> w1813
                                tunnel: [w1909] -> w1812
                                tunnel: w1813 -> [w1919]
                                tunnel: w1812 -> [w1918]
                                tunnel: [w1919] -> w1811
                                tunnel: [w1918] -> w1810
                                tunnel: [w1921] -> w1814
                                tunnel: [w1922] -> w1817
                                tunnel: w1811 -> [w1922]
                                tunnel: w1810 -> [w1921]
                                frame #0 {
                                n1592 = local read "SC measured test time hid"() -> (w1826:dbl)
                                n1593 = local read "SC measured wait time hid"() -> (w1827:dbl)
                                n1594 = Add(x=w1826, y=w1827) -> (x+y=w1833:dbl)
                                n1595 = local read "Tester loop counter hid"() -> (w1829:u32)
                                n1596 = local read "Utilization averaging"() -> (w1828:i32)
                                n1597 = Divide(x=w1826, y=w1833) -> (x/y=w1834:dbl)
                                n1598 = Multiply(x=100.0, y=w1834) -> (x*y=w1830:dbl)
                                n1599 = call "moving_avg_core.vi"("Array in"=w1824, "avg"=w1828, "accumulator in"=w1825, "i"=w1829, "data in"=w1830) -> ("Array out"=w1823:dbl[], "accumulator out"=w1822:dbl, "rolling avg out"=w1831:dbl)  [unwired: 4 in]
                                n1600 = local write "Sys utilization"(w1831) -> ()
                                n1601 = Bundle(w1830, "rolling avg out"=w1831) -> (w1832:cluster{dbl, "rolling avg out":dbl})  [unwired: 1 in]
                                n1602 = local write "SysUtilMon"(w1832) -> ()
                                }
                                frame #1 {
                                # "This is the engine that decides if H1 is checked first or H2"
                                n1603 = local read "Last locked handler hid"() -> (w1836:enum16{"H1", "H2"})
                                n1604 = case shown="\"H1\", Default" w1836 {
                                frame "H1", Default {
                                n1605 = local read "H2 Ready with sites"() -> (w1839:bool)
                                n1606 = case shown="False" w1839 {
                                frame False {
                                n1607 = local read "H1 Ready with sites"() -> (w1840:bool)
                                n1608 = case shown="True" w1840 {
                                frame False {
                                # "end up here only if neither handler is waiting and ready"
                                }
                                frame True {
                                n1609 = flat-sequence {
                                frame #0 {
                                n1610 = local write "H1 Lock"(TRUE ("H1 Lock")) -> ()
                                n1611 = local write "H2 Lock"(FALSE ("H1 Lock")) -> ()
                                n1612 = local write "Last locked handler hid"(enum16{"H1", "H2"}."H1" ("Last locked handler")) -> ()
                                }
                                frame #1 {
                                n1613 = while {
                                stop <- w1844 stop-if-true
                                n1614 = local read "VISA bus 0 resource name out hid"() -> (w1853:refnum<visa-resource-name>)
                                n1615 = local read "H1 SITES? response hid"() -> (w1847:string)
                                n1616 = local read "VISA bus 0 error out hid"() -> (w1854:errorcluster)
                                n1617 = VISA Write(VISA resource name=w1853, write buffer=w1847, error in (no error)=w1854) -> (VISA resource name out=w1852:refnum<visa-resource-name>, return count=w1845:u32, error out=w1851:errorcluster)
                                n1618 = local write "VISA bus 0 resource name out hid"(w1852) -> ()
                                n1619 = local write "VISA bus 0 error out hid"(w1851) -> ()
                                n1620 = Unbundle By Name(w1851) -> ("status"=w1855:bool)
                                n1621 = Concatenate Strings("H1: Tester test cycle start" ("string"), "\r\n", "Bus 0 write: " ("string"), w1847) -> (w1849:string)
                                n1622 = Greater Than 0?(x=w1845) -> (x > 0?=w1844:bool)
                                n1623 = local write "GPIB bus 0 write error"(w1855) -> ()
                                n1624 = local write "GPIB Bus 0 traffic"(w1849) -> ()
                                }
                                }
                                frame #2 {
                                n1625 = local read "H1 loop counter hid"() -> (w1857:u32)
                                n1626 = Increment(x=w1857) -> (x+1=w1856:u32)
                                n1627 = local write "H1 loop counter hid"(w1856) -> ()
                                }
                                }
                                }
                                }
                                }
                                frame True {
                                n1628 = flat-sequence {
                                frame #0 {
                                n1629 = local write "H2 Lock"(TRUE ("H1 Lock")) -> ()
                                n1630 = local write "H1 Lock"(FALSE ("H1 Lock")) -> ()
                                n1631 = local write "Last locked handler hid"(enum16{"H1", "H2"}."H2" ("Last locked handler")) -> ()
                                }
                                frame #1 {
                                n1632 = while {
                                stop <- w1862 stop-if-true
                                n1633 = local read "VISA bus 0 resource name out hid"() -> (w1870:refnum<visa-resource-name>)
                                n1634 = local read "H2 SITES? response hid"() -> (w1864:string)
                                n1635 = local read "VISA bus 0 error out hid"() -> (w1871:errorcluster)
                                n1636 = VISA Write(VISA resource name=w1870, write buffer=w1864, error in (no error)=w1871) -> (VISA resource name out=w1869:refnum<visa-resource-name>, return count=w1861:u32, error out=w1868:errorcluster)
                                n1637 = local write "VISA bus 0 resource name out hid"(w1869) -> ()
                                n1638 = local write "VISA bus 0 error out hid"(w1868) -> ()
                                n1639 = Unbundle By Name(w1868) -> ("status"=w1872:bool)
                                n1640 = Concatenate Strings("H2: Tester test cycle start" ("string"), "\r\n", "Bus 0 write: " ("string"), w1864) -> (w1866:string)
                                n1641 = Greater Than 0?(x=w1861) -> (x > 0?=w1862:bool)
                                n1642 = local write "GPIB bus 0 write error"(w1872) -> ()
                                n1643 = local write "GPIB Bus 0 traffic"(w1866) -> ()
                                }
                                }
                                frame #2 {
                                n1644 = local read "H2 loop counter hid"() -> (w1873:u32)
                                n1645 = Increment(x=w1873) -> (x+1=w1874:u32)
                                n1646 = local write "H2 loop counter hid"(w1874) -> ()
                                }
                                }
                                }
                                }
                                }
                                frame "H2" {
                                n1647 = local read "H1 Ready with sites"() -> (w1875:bool)
                                n1648 = case shown="True" w1875 {
                                frame False {
                                n1649 = local read "H2 Ready with sites"() -> (w1876:bool)
                                n1650 = case shown="True" w1876 {
                                frame False {
                                # "end up here only if neither handler is waiting and ready"
                                }
                                frame True {
                                n1651 = flat-sequence {
                                frame #0 {
                                n1652 = local write "H1 Lock"(FALSE ("H1 Lock")) -> ()
                                n1653 = local write "H2 Lock"(TRUE ("H1 Lock")) -> ()
                                n1654 = local write "Last locked handler hid"(enum16{"H1", "H2"}."H2" ("Last locked handler")) -> ()
                                }
                                frame #1 {
                                n1655 = while {
                                stop <- w1881 stop-if-true
                                n1656 = local read "VISA bus 0 resource name out hid"() -> (w1889:refnum<visa-resource-name>)
                                n1657 = local read "H2 SITES? response hid"() -> (w1883:string)
                                n1658 = local read "VISA bus 0 error out hid"() -> (w1890:errorcluster)
                                n1659 = VISA Write(VISA resource name=w1889, write buffer=w1883, error in (no error)=w1890) -> (VISA resource name out=w1888:refnum<visa-resource-name>, return count=w1880:u32, error out=w1887:errorcluster)
                                n1660 = local write "VISA bus 0 resource name out hid"(w1888) -> ()
                                n1661 = local write "VISA bus 0 error out hid"(w1887) -> ()
                                n1662 = Unbundle By Name(w1887) -> ("status"=w1891:bool)
                                n1663 = Concatenate Strings("H2: Tester test cycle start" ("string"), "\r\n", "Bus 0 write: " ("string"), w1883) -> (w1885:string)
                                n1664 = Greater Than 0?(x=w1880) -> (x > 0?=w1881:bool)
